vi "ExSubCreateData.vi"(2 "error in (no error)":errorcluster, 3 "File and Display Name":string, 4 "Pulser Handle":u32, 5 "Camera Handle":u32) -> (0 "error out":errorcluster, 1 "Handles Out":T1)   [LabVIEW 2010]
panel:
  # "ExSubCreateData:\nThis is a SubVI that creates image objects and returns the handles bundled in a cluster that includes a pulser and camera handle"
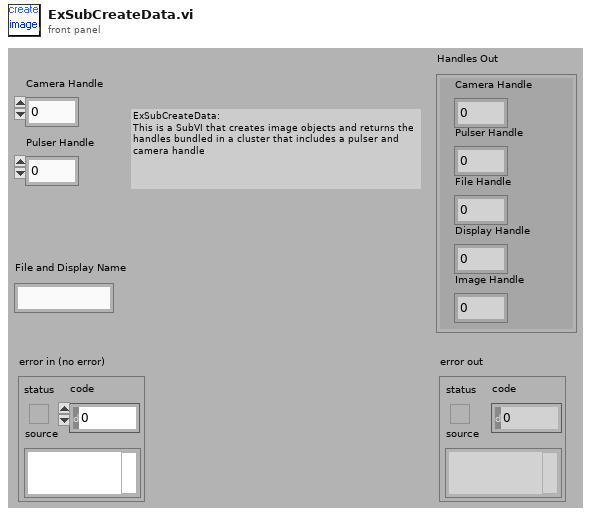
[diagram p1: front panel]
types:
  T1 = cluster{"Camera Handle":u32, "Pulser Handle":u32, "File Handle":u32, "Display Handle":u32, "Image Handle":u32}
  T2 = cluster{"Camera Handle":u32, "Pulser Handle":u32, i32, i32, "Image Handle":u32}
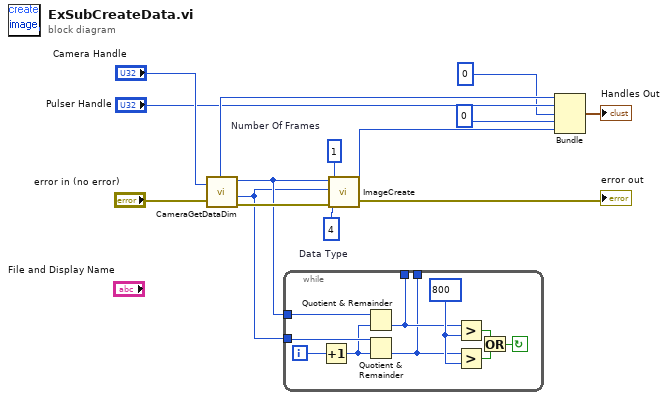
[diagram p0: block diagram]
diagram:
  w7 = u32 1  # Number Of Frames
  w8 = u32 4  # Data Type
  n1 = call <userlib>:"CameraGetDataDim.vi"("Camera Handle"="Camera Handle", "error in"="error in (no error)") -> ("Camera Handle"=w11:u32, "Xdim"=w6:u32, "Ydim"=w5:u32, "error out"=w14:errorcluster)
  n2 = while {
    tunnel: w6 -> [w23]
    tunnel: w5 -> [w22]
    tunnel: [w17] -> _
    tunnel: [w16] -> _
    i -> [w21]
    stop <- w18 continue-if-true
    w24 = 800
    n3 = Increment(x=w21) -> (x+1=w15:i32)
    n4 = Quotient & Remainder(x=w23, y=w15) -> (floor(x/y)=w17:u32)  [unwired: 1 out]
    n5 = Quotient & Remainder(x=w22, y=w15) -> (floor(x/y)=w16:u32)  [unwired: 1 out]
    n6 = Greater?(x=w17, y=w24) -> (0:w20:bool)
    n7 = Greater?(x=w16, y=w24) -> (0:w19:bool)
    n8 = Or(x=w20, y=w19) -> (x .or. y?=w18:bool)
  }
  n9 = call <userlib>:"ImageCreate.vi"("X dimension"=w6, "Y dimension"=w5, "Data Type"=w8, "error in"=w14, "Number Of Frames"=w7) -> ("Image Handle"=w9:u32, "error out"=→"error out":errorcluster)
  n10 = Bundle("Camera Handle"=w11, "Pulser Handle"="Pulser Handle", 0, 0, "Image Handle"=w9) -> (→"Handles Out":T2)  [unwired: 1 in]
